vi "DataLog Test Base Tag Validity.vi"(7 "base tag":string, 11 "error in (no error)":errorcluster) -> (8 "base tag dup":string, 15 "error out":errorcluster)   [LabVIEW 2012]
doc: "Tests if the provided tag is a valid tag for a non-meta tag."
uses:
  typedefs/t_DataLog Tag Expression Evaluator Methods.ctl
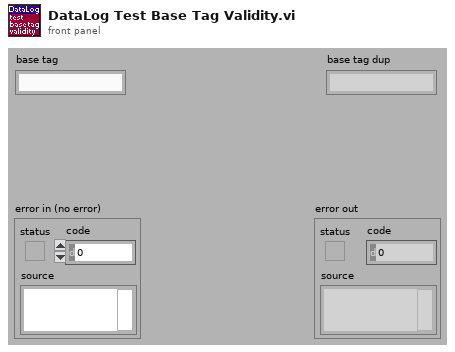
[diagram p1: front panel]
types:
  T1 = typedef "t_DataLog Tag Expression Evaluator Methods.ctl" = enum16{"set", "get", "eval", "assign", "execute", "isvalid", "clear"}
  T2 = typedef "et_DataLog Meta Tag Specifier.ctl" = enum32{"warn_lo", "warn_hi", "A_lo", "A_hi", "B_lo", "B_hi", "C_lo", "C_hi", "D_lo", "D_hi", "E_lo", "E_hi", "F_lo", "F_hi", "G_lo", "G_hi", "H_lo", "H_hi", "I_lo", "I_hi", "J_lo", "J_hi", "K_lo", "K_hi", "L_lo", "L_hi", "M_lo", "M_hi", "N_lo", "N_hi", "min", "max", "not a meta"}
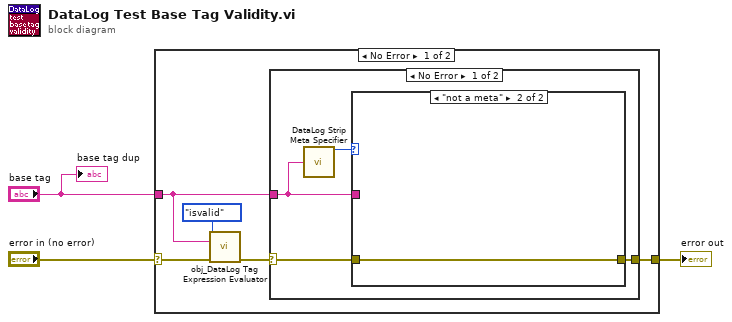
[diagram p0: block diagram]
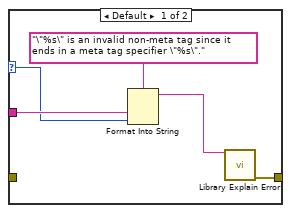
[diagram p2: hidden frame]
diagram:
  n1 = case shown="No Error" "error in (no error)" {
    selector: "error in (no error)" -> [w7 w20]
    tunnel: [w8 w20] -> w3
    tunnel: "base tag" -> [w5 _]
    frame No Error {
      n2 = call "obj_DataLog Tag Expression Evaluator.vi"("method"=t_DataLog_Tag_Expression_Evaluator_Methods."isvalid", "variable"=w5, "error in (no error)"=w7) -> ("error out"=w4:errorcluster)  [unwired: 11 in, 1 out]
      n3 = case shown="No Error" w4 {
        selector: w4 -> [w12 w19]
        tunnel: w5 -> [w10 _]
        tunnel: [w11 w19] -> w8
        frame No Error {
          n4 = call "DataLog Strip Meta Specifier.vi"("tag"=w10) -> ("meta specifier"=w9:T2)  [unwired: 13 in, 1 out]
          n5 = case shown="\"not a meta\"" w9 {
            selector: w9 -> [w13 _]
            tunnel: [w16 w18] -> w11
            tunnel: w12 -> [_ w18]
            tunnel: w10 -> [w17 _]
            frame Default {
              n6 = Format Into String(format string="\"%s\" is an invalid non-meta tag since it ends in a meta tag specifier \"%s\".", w17, w13) -> (resulting string=w15:string)  [unwired: 2 in, 1 out]
              n7 = call "Library Explain Error.vi"("explanation prefix (none)"=w15) -> ("explained error"=w16:errorcluster)  [unwired: 14 in]
            }
            frame "not a meta" {
            }
          }
        }
        frame Error {
        }
      }
    }
    frame Error {
    }
  }
  "error out" <- w3
  "base tag dup" <- "base tag"
